vi "LSX Set Hw Factor Single Axis.vi"(8 "error in (no error)":errorcluster, 9 "dFactor":dbl, 10 "lAxis":i32, 11 "lLSID":i32) -> (0 "error out":errorcluster, 3 "function return":i32)   [LabVIEW 2018, in "Tango.lvlib"]
doc: "TANGOAPI int TANGOCALL LSX_SetHwFactorSingleAxis (int lLSID, int lAxis, double dFactor);"
uses:
  Tango.lvlib
  SubVIs/Tango_DLL.dll
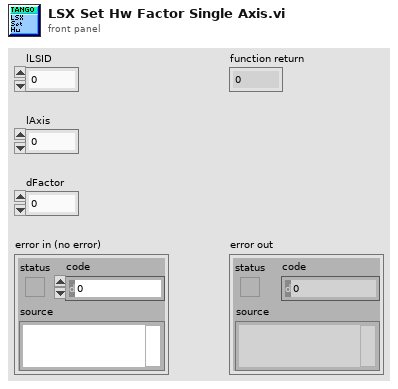
[diagram p1: front panel]
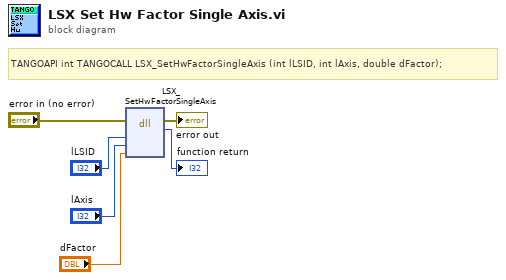
[diagram p0: block diagram]
diagram:
  # "TANGOAPI int TANGOCALL LSX_SetHwFactorSingleAxis (int lLSID, int lAxis, double dFactor);"
  n1 = dll-call lib="C:/Users/Familie/Documents/LabviewIX81/lib/TANGO Stage/SubVIs/Tango_DLL.*" fn="LSX_SetHwFactorSingleAxis"(error in="error in (no error)", "lLSID"="lLSID", "lAxis"="lAxis", "dFactor"="dFactor") -> (error out=→"error out":errorcluster, →"function return":i32)  [unwired: 5 in, 1 out]
